vi "thing.vi"(11 "String":string) -> (3 "Array":string[](array[string]))   [LabVIEW 2017]
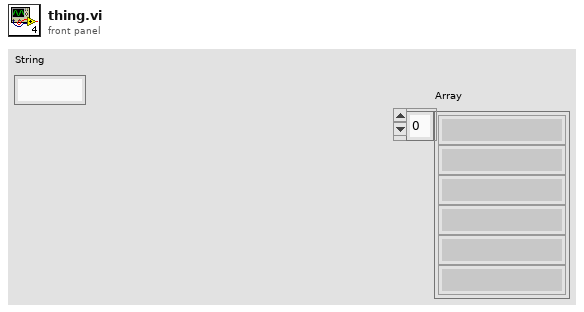
[diagram p1: front panel]
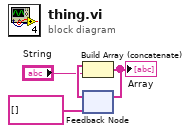
[diagram p0: block diagram]
diagram:
  n1 = feedback #1(string[] [] ("Array")) -> (w3:string[])
  n2 = Build Array (concatenate)(w3, "String") -> (w1:string[])
  "Array" <- w1
  n3 = feedback-in #1(w1) -> ()
